vi "To BananaLeaf.TestCase.vi"(10 "Properties.Test":refnum<class "Properties.Test.lvclass">) -> (3 "Leaf.Properties.TestCase out":refnum<class "Leaf.Properties.Test.lvclass">)   [LabVIEW 2021, in "Banana.Caraya.lvlib" / "Leaf.Properties.Test.lvclass"]
uses:
  Leaf.Properties.Test.lvclass
  C:/Repositories/LVOS/Bananas/lv-src/Banana.Caraya/Leaf.Properties/Leaf.Properties.lvclass
  Leaf.Properties/Leaf.Properties.lvclass/Leaf.Properties.ctl
  Leaf.Properties.Test.lvclass/Leaf.Properties.Test.ctl
  Leaf.Properties/Leaf.Properties.lvclass
  <vilib>/addons/_JKI Toolkits/Caraya/classes/Properties.Test/Properties.Test.lvclass
  C:/Program Files (x86)/National Instruments/LabVIEW 2021/vi.lib/addons/_JKI Toolkits/Caraya/classes/Properties/Properties.lvclass
  C:/Program Files (x86)/National Instruments/LabVIEW 2021/vi.lib/addons/_JKI Toolkits/Caraya/classes/Properties.Test/Properties.Test.lvclass
  C:/Repositories/LVOS/Bananas/lv-src/Bananas/Leaf/Leaf.lvclass
  C:/Repositories/LVOS/Bananas/lv-src/Bananas/Leaf.TestCase/Leaf.TestCase.lvclass
  C:/Repositories/LVOS/Bananas/lv-src/Banana.Caraya/Leaf.Properties.Test/Leaf.Properties.Test.lvclass
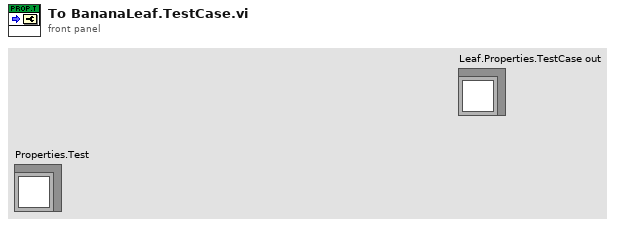
[diagram p1: front panel]
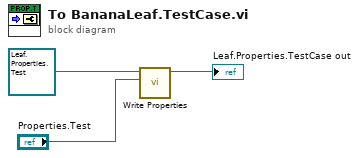
[diagram p0: block diagram]
diagram:
  n1 = call "Write Properties.vi"("Properties"="Properties.Test", "Leaf.Properties in"=refnum<class "Leaf.Properties.Test.lvclass"> refnum ("Leaf.Properties.Assert in")) -> ("Leaf.Properties out"=→"Leaf.Properties.TestCase out":refnum<class "Leaf.Properties.Test.lvclass">)  [unwired: 9 in]
